vi "dosimat876_execute_method.vi"(2 "error in":errorcluster, 3 "Dosimat Port In":refnum<visa-resource-name>="COM1") -> (0 "error out":errorcluster, 1 "Dosimat Port Out":refnum<visa-resource-name>="COM1")   [LabVIEW 2010]
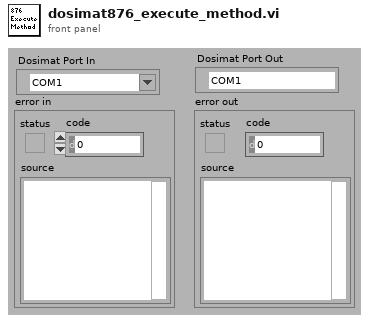
[diagram p1: front panel]
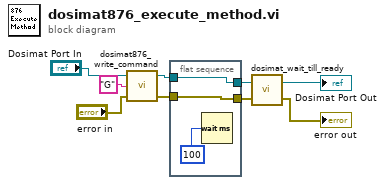
[diagram p0: block diagram]
diagram:
  n1 = call "dosimat876_write_command.vi"("error in"="error in", "write buffer"="G", "Dosimat Port In"="Dosimat Port In") -> ("error out"=w1:errorcluster, "Dosimat Port Out"=w3:refnum<visa-resource-name>)  [unwired: 1 out]
  n2 = flat-sequence {
    tunnel: [w11] -> w4
    tunnel: w3 -> [w11]
    tunnel: [w10] -> w2
    tunnel: w1 -> [w10]
    frame #0 {
      n3 = Wait (ms)(milliseconds to wait=100) -> ()  [unwired: 1 out]
    }
  }
  n4 = call "dosimat_wait_till_ready.vi"("error in"=w2, "Dosimat Port In"=w4) -> ("error out"=→"error out":errorcluster, "Dosimat Port Out"=→"Dosimat Port Out":refnum<visa-resource-name>)
